vi "Mask Write Register.vi"(4 "OR mask":u16, 6 "AND mask":u16=65535, 8 "error in (no error)":errorcluster, 10 "address":u16, 11 "device data model in":refnum<class "ICPCON ET Data Model.lvclass">) -> (0 "error out":errorcluster, 3 "device data model out":refnum<class "ICPCON ET Data Model.lvclass">)   [LabVIEW 2021, in "ICPCON ET Data Model.lvclass"]
doc: "Writes the masked value of a single register using an <b>AND mask</b> and an <b>OR mask</b> using the equation below:\nResult=(Current Value AND AndMask) OR (OrMask AND !AndMask)"
uses:
  ICPCON ET Data Model.lvclass
  ICPCON ET Data Model.lvclass/ICPCON ET Data Model.ctl
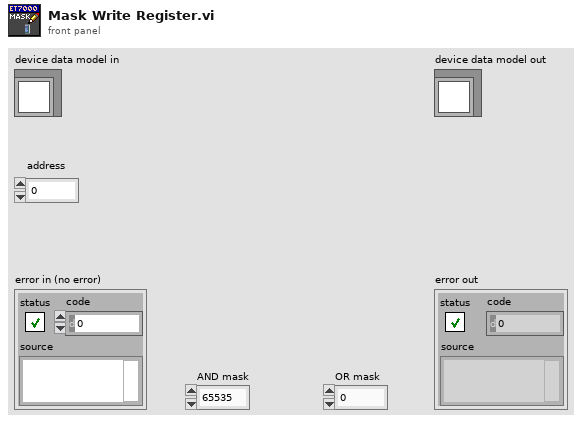
[diagram p1: front panel]
types:
  T1 = typedef "ICPCON ET Data Model.lvclass/Data Model.ctl" = cluster{"UTC":u64, "DI":bool[], "DO":bool[], "IR":u16[], "HR":u16[], "ES":u8}
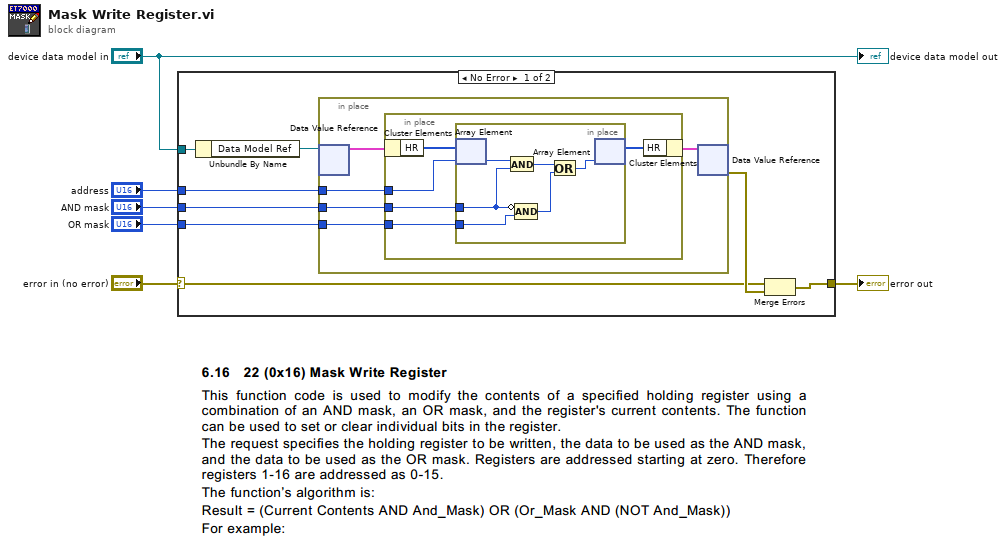
[diagram p0: block diagram]
diagram:
  n1 = case shown="No Error" "error in (no error)" {
    selector: "error in (no error)" -> [w7 w31]
    tunnel: "device data model in" -> [w14 _]
    tunnel: [w13 w31] -> w5
    tunnel: "address" -> [w12 _]
    tunnel: "AND mask" -> [w11 _]
    tunnel: "OR mask" -> [w10 _]
    frame No Error {
      n2 = Unbundle By Name(w14) -> ("Data Model Ref"=w9:refnum<data-value>)
      n3 = in-place {
        in-place-border: w12 -> [w19]
        in-place-border: w11 -> [w18]
        in-place-border: w10 -> [w17]
        n4 = in-place-dvr #1(w9) -> (w15:T1)  [unwired: 1 out]
        n5 = in-place {
          in-place-border: w19 -> [w24]
          in-place-border: w18 -> [w23]
          in-place-border: w17 -> [w22]
          n6 = in-place-cluster #2(w15) -> ("HR"=w21:u16[])
          n7 = in-place {
            in-place-border: w23 -> [w27]
            in-place-border: w22 -> [w25]
            n8 = in-place-array #3(w21, w24) -> (w26:u16)
            n9 = And(x=w26, y=w27) -> (x .and. y?=w29:u16)
            n10 = Compound Arithmetic op=AND(invert w27, w25) -> (w30:u16)
            n11 = Or(x=w29, y=w30) -> (x .or. y?=w28:u16)
            n12 = in-place-array #3(w28) -> (w20:u16[])  [unwired: 1 out]
          }
          n13 = in-place-cluster #2("HR"=w20) -> (w16:T1)
        }
        n14 = in-place-dvr #1(w16) -> (w8:errorcluster)  [unwired: 1 out]
      }
      n15 = Merge Errors(w7, w8) -> (w13:errorcluster)
    }
    frame Error {
    }
  }
  "error out" <- w5
  "device data model out" <- "device data model in"
